vi "Clear.vi"(8 "error in (no error)":errorcluster, 11 "Store in":refnum<class "Store.lvclass">) -> (0 "error out":errorcluster, 3 "Store out":refnum<class "Store.lvclass">)   [LabVIEW 2018, in "Application.lvlib" / "Store.lvclass"]
uses:
  Store.lvclass
  Store.lvclass/Store.ctl
  Dictionary Class/Dictionary.lvclass/Dictionary.ctl
  Dictionary Class/VIs/Get Data DVR.vi
  Dictionary Class/Dictionary.lvclass
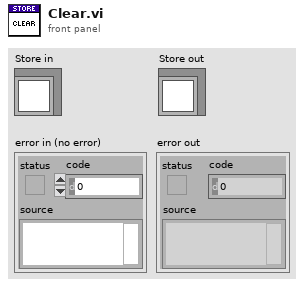
[diagram p1: front panel]
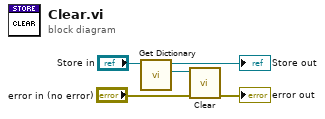
[diagram p0: block diagram]
diagram:
  n1 = call "Get Dictionary.vi"("Store in"="Store in") -> ("Dictionary.lvclass"=w4:refnum<class "Dictionary.lvclass">, "Store out"=→"Store out":refnum<class "Store.lvclass">)  [unwired: 8 in, 1 out]
  n2 = call "Clear.vi"("error in (no error)"="error in (no error)", "Dictionary in"=w4) -> ("error out"=→"error out":errorcluster)  [unwired: 8 in, 1 out]
